vi "InitRingValue.vi"(8 "ErrorArray In":errorcluster[](array[cluster]), 10 "RingRefArray":refnum<vi>[](array[refnum]), 11 "IniFileRef":T1) -> (0 "ErrorArray Out":errorcluster[](array[cluster]), 3 "IniFileRef out":T1)   [LabVIEW 2014, in "Ini_lib.lvlib"]
uses:
  Ini_lib.lvlib
  <vilib>/Utility/config.llb/Config Data RefNum.ctl
  <vilib>/Utility/config.llb/Read Key (String).vi
  <vilib>/Utility/config.llb/NI_LVConfig.lvlib
  <userlib>/NIST/NISTErrorLib/NISTErrorLib.lvlib
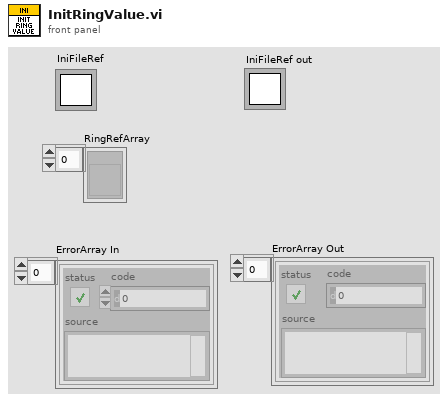
[diagram p1: front panel]
types:
  T1 = typedef "NI_LVConfig.lvlib/Config Data RefNum.ctl" = refnum<k1>
  T2 = typedef "LVStringsAndValuesArrayTypeDef_U16.ctl" = cluster{"String":string, "Value":u16}[]
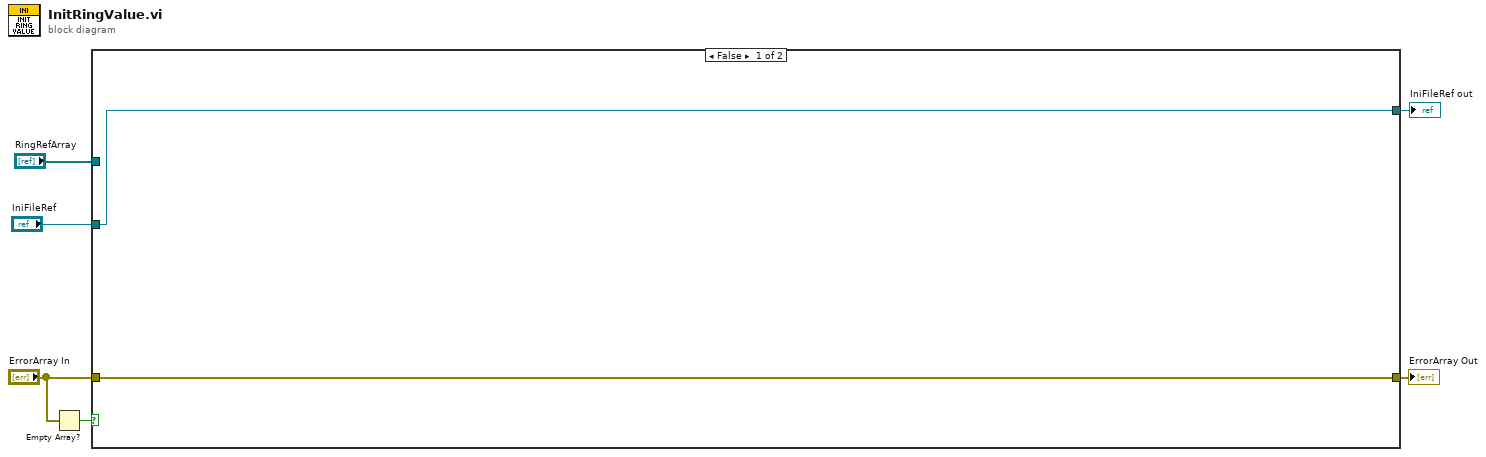
[diagram p0: block diagram]
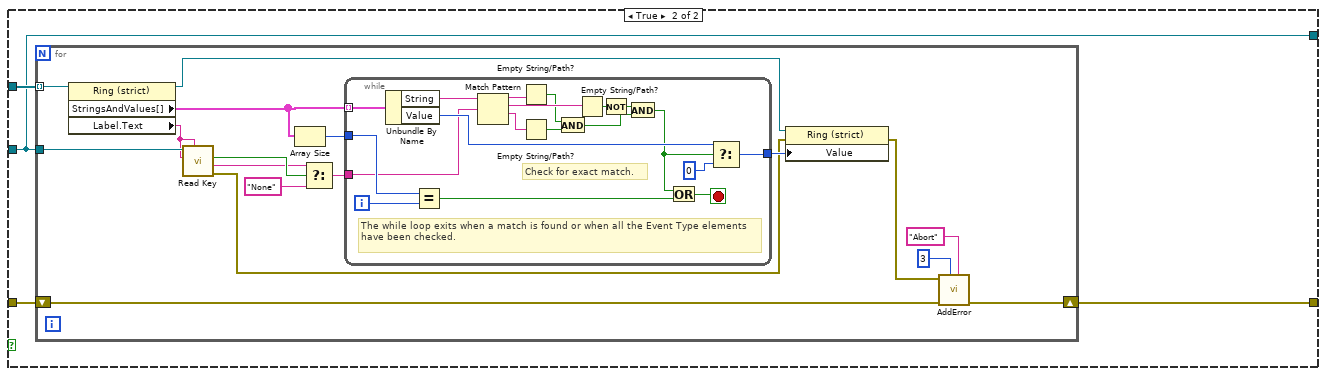
[diagram p2: hidden frame]
diagram:
  n1 = Empty Array?(array="ErrorArray In") -> (empty?=w6:bool)
  n2 = case shown="False" w6 {
    tunnel: "ErrorArray In" -> [w8 w12]
    tunnel: [w8 w11] -> w4
    tunnel: "IniFileRef" -> [w7 w9]
    tunnel: "RingRefArray" -> [_ w10]
    tunnel: [w7 w9] -> w1
    frame False {
    }
    frame True {
      n3 = for {
        tunnel: w10 -> [w14] mode=indexing
        tunnel: w9 -> [w29]
        shift-right: [w16] -> w11
        shift-left: w12 -> [w17]
        n4 = property class="Ring (strict)"(reference=w14) -> (reference out=w13:refnum<vi>, "StringsAndValues[]"=w27:T2, "Label.Text"=w15:string)  [unwired: 1 in, 1 out]
        n5 = call-poly <vilib>:"Read Key.vi"("section"=w15, "key"=w15, "refnum"=w29) -> ("error out"=w21:errorcluster, "value"=w23:string, "found?"=w24:bool)  [unwired: 5 in, 1 out]
        n6 = Array Size(array=w27) -> (size(s)=w26:i32)
        n7 = Select(t=w23, s=w24, f="None" ("regular expression")) -> (s? t:f=w22:string)
        n8 = while {
          tunnel: w27 -> [w36] mode=indexing
          tunnel: [w32] -> w28
          tunnel: w26 -> [w31]
          tunnel: w22 -> [w30]
          i -> [w39]
          stop <- w38 stop-if-true
          # "The while loop exits when a match is found or when all the Event Type elements have been checked."
          # "Check for exact match."
          n9 = Unbundle By Name(w36) -> ("String"=w48:string, "Value"=w35:u16)
          n10 = Equal?(x=w31, y=w39) -> (x = y?=w37:bool)
          n11 = Match Pattern(string=w48, regular expression=w30) -> (before substring=w45:string, match substring=w47:string, after substring=w44:string)  [unwired: 1 in, 1 out]
          n12 = Empty String/Path?(string/path=w45) -> (empty?=w42:bool)
          n13 = Empty String/Path?(string/path=w44) -> (empty?=w43:bool)
          n14 = And(x=w42, y=w43) -> (x .and. y?=w41:bool)
          n15 = Empty String/Path?(string/path=w47) -> (empty?=w46:bool)
          n16 = Not(x=w46) -> (.not. x?=w40:bool)
          n17 = And(x=w40, y=w41) -> (x .and. y?=w33:bool)
          n18 = Or(x=w33, y=w37) -> (x .or. y?=w38:bool)
          n19 = Select(t=w35, s=w33, f=u16 0) -> (s? t:f=w32:u16)
        }
        n20 = property class="Ring (strict)"(reference=w13, error in=w21, "Value"=w28) -> (error out=w20:errorcluster)  [unwired: 1 out]
        n21 = call <userlib>:"AddError.vi"("Severity"="Abort", "Priority"=u8 3, "ErrorArray"=w17, "error in (no error)"=w20) -> ("ErrorArray"=w16:errorcluster[])  [unwired: 6 in, 1 out]
      }
    }
  }
  "ErrorArray Out" <- w4
  "IniFileRef out" <- w1
